vi "macro_Ctrl_LTVUnicycleExecute.vi"() -> ()   [LabVIEW 2019]
uses:
  <vilib>/Rock Robotics/WPI/ThirdParty/JAS_Junk/TrajLib/Trajectory_Library.lvlib
  <vilib>/Rock Robotics/WPI/ThirdParty/JAS_Junk/TrajLib/TypeDef/TRANSLATION2D.ctl
  <vilib>/Rock Robotics/WPI/ThirdParty/JAS_Junk/TrajLib/TypeDef/ROTATION2D.ctl
  <vilib>/Rock Robotics/WPI/ThirdParty/JAS_Junk/TrajLib/TypeDef/POSE2D.ctl
  TypeDef/PathPlannerPathConstraints.ctl
  TypeDef/PathPlannerTrajectoryState.ctl
panel:
  in  "CurrentPose":T1={"TRANSLATION"={"X"=0.0, "Y"=0.0}, "ROTATION"={"VALUE"=0.0, "COS"=1.0, "SIN"=0.0}} {"ROTATION"."SIN" format="%13.4f"; "ROTATION"."COS" format="%13.4f"; "ROTATION"."VALUE" format="%13.4f"; "TRANSLATION"."Y" format="%14.3f"; "TRANSLATION"."X" format="%14.3f"}
  out "Right Speed Dmd M/S":dbl
  out "Left Speed Dmd M/S":dbl
  in  "PathPlannerState":T4={"TimeSeconds"=0.0, "VelocityMPS"=0.0, "AccerationMpsSq"=0.0, "HeadingAngularVelRadPerSec"=0.0, "PositionMeters"={"X"=0.0, "Y"=0.0}, "Heading"={"VALUE"=0.0, "COS"=1.0, "SIN"=0.0}, "TargetHolonomicRotation"={"VALUE"=0.0, "COS"=1.0, "SIN"=0.0}, "CurvatureRadPerMeter"=0.0, "PathPlannerConstraints"={"MaxVelocityMps;"=0.0, "MaxAccelerationMpsSq;"=0.0, "MaxAngularVelRadPsEc;"=0.0, "MaxAngularAccRadPSecSq"=0.0, "Exists"=FALSE}, "DeltaPos"=0.0} {"TargetHolonomicRotation"."SIN" format="%13.4f"; "TargetHolonomicRotation"."COS" format="%13.4f"; "TargetHolonomicRotation"."VALUE" format="%13.4f"; "Heading"."SIN" format="%13.4f"; "Heading"."COS" format="%13.4f"; "Heading"."VALUE" format="%13.4f"; "PositionMeters"."Y" format="%14.3f"; "PositionMeters"."X" format="%14.3f"}
  out "Position Error M":dbl
  out "At Reference":bool
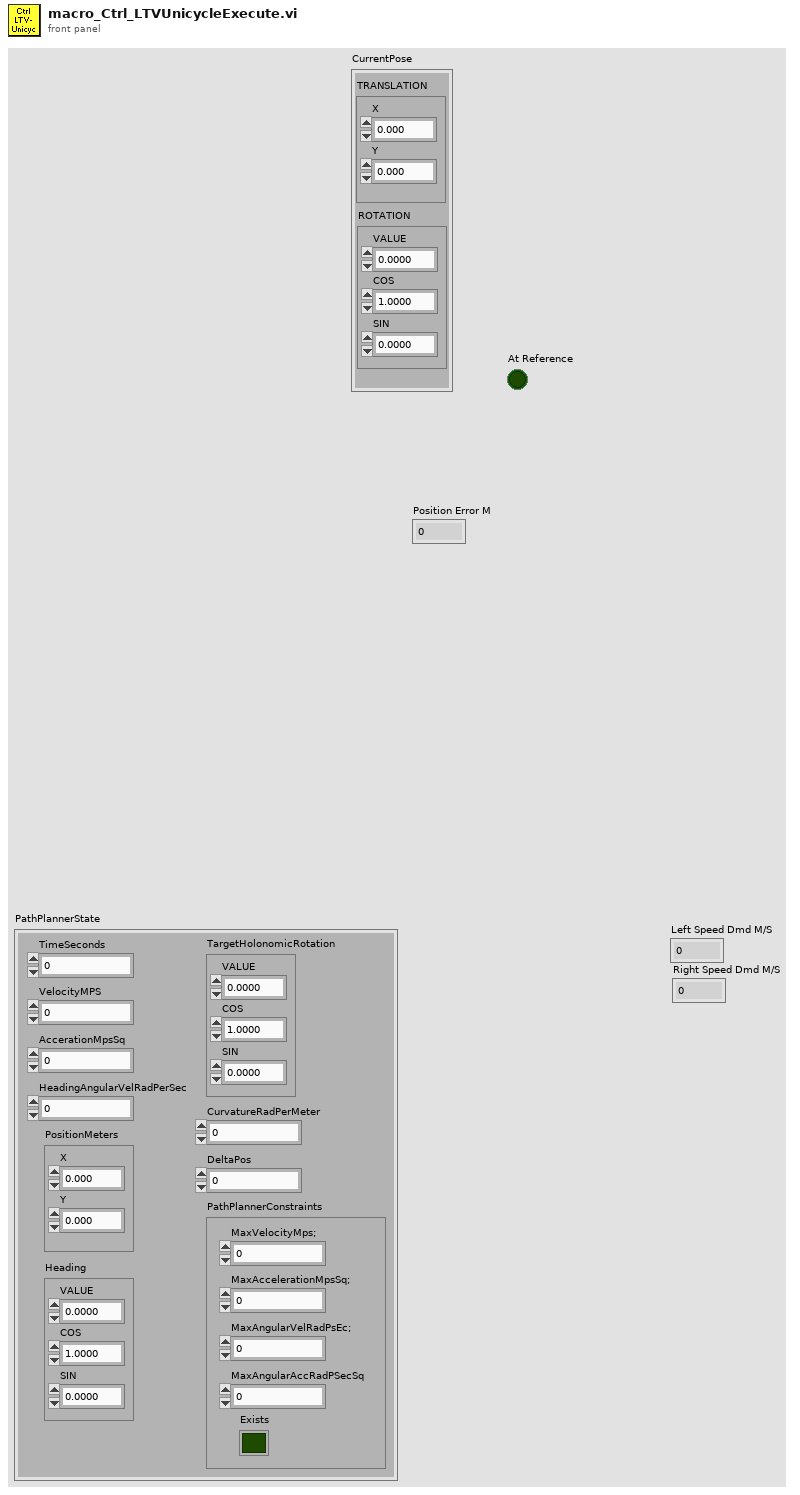
[diagram p1: front panel]
types:
  T1 = typedef "Trajectory_Library.lvlib/POSE2D.ctl" = cluster{"TRANSLATION":T2, "ROTATION":T3}
  T2 = typedef "Trajectory_Library.lvlib/TRANSLATION2D.ctl" = cluster{"X":dbl, "Y":dbl}
  T3 = typedef "Trajectory_Library.lvlib/ROTATION2D.ctl" = cluster{"VALUE":dbl, "COS":dbl, "SIN":dbl}
  T4 = typedef "PathPlannerTrajectoryState.ctl" = cluster{"TimeSeconds":dbl, "VelocityMPS":dbl, "AccerationMpsSq":dbl, "HeadingAngularVelRadPerSec":dbl, "PositionMeters":T2, "Heading":T3, "TargetHolonomicRotation":T3, "CurvatureRadPerMeter":dbl, "PathPlannerConstraints":T5, "DeltaPos":dbl}
  T5 = typedef "PathPlannerPathConstraints.ctl" = cluster{"MaxVelocityMps;":dbl, "MaxAccelerationMpsSq;":dbl, "MaxAngularVelRadPsEc;":dbl, "MaxAngularAccRadPSecSq":dbl, "Exists":bool}
  T6 = typedef "Trajectory_Library.lvlib/LTV_UNICYCLE_CONTROLLER_MODEL_PARAMS.CTL" = cluster{"Max linear ctrl effort M/S":dbl, "Max angular ctrl effort Rad/S":dbl, "Max Heading Meas Tol Rad":dbl, "Max X Pos Meas Tol M":dbl, "Max Y Pos Meas Tol M":dbl, "Max Linear Vel M/S":dbl}
  T7 = typedef "PathPlannerCtrlLTVUnicycleConfig.ctl" = cluster{"Max Wheel Speed M/S":dbl, "Track Width M":dbl, "LTV_Unicycle_Ctrl_Model":T6, "LTV_Unicycle_Ctrl_Tolerance":T8}
  T8 = typedef "Trajectory_Library.lvlib/LTV_UNICYCLE_CONTROLLER_TOLERANCE.CTL" = cluster{"Max Heading Tolerance Rad":dbl, "Max X Tolerance M":dbl, "Max Y Tolerance M":dbl}
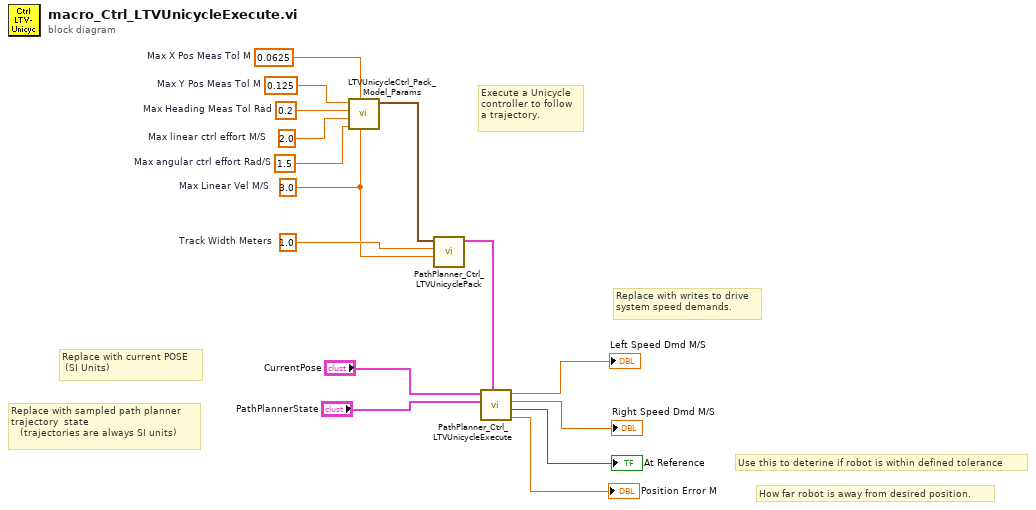
[diagram p0: block diagram]
diagram:
  w2 = 1.0  # Track Width Meters
  w11 = 0.125  # Max Y Pos Meas Tol M
  w12 = 0.2  # Max Heading Meas Tol Rad
  w13 = 2.0  # Max linear ctrl effort M/S
  w14 = 1.5  # Max angular ctrl effort Rad/S
  w15 = 0.0625  # Max X Pos Meas Tol M
  w1 = 3.0  # Max Linear Vel M/S
  # "Execute a Unicycle\ncontroller to follow\na trajectory."
  # "Replace with writes to drive\nsystem speed demands."
  # "Replace with current POSE\n (SI Units)"
  # "Replace with sampled path planner \ntrajectory  state \n   (trajectories are always SI units)"
  # "How far robot is away from desired position."
  # "Use this to deterine if robot is within defined tolerance"
  n1 = call <vilib>:"LTVUnicycleCtrl_Pack_Model_Params.vi"("Max Linear Vel M/S"=w1, "Max X Pos Meas Tol M"=w15, "Max angular ctrl effort Rad/S"=w14, "Max linear ctrl effort M/S"=w13, "Max Heading Meas Tol Rad"=w12, "Max Y Pos Meas Tol M"=w11) -> ("LTV_Unicycle_Ctrl_Model _Params"=w3:T6)  [unwired: 5 in]
  n2 = call "PathPlanner_Ctrl_LTVUnicyclePack.vi"("Max Speed M/S"=w1, "Track Width Meters"=w2, "LTV_Unicycle_Ctrl_Model"=w3) -> ("PathPlanner_Ctrl_LTVUnicycleConfig"=w4:T7)  [unwired: 8 in]
  n3 = call "PathPlanner_Ctrl_LTVUnicycleExecute.vi"("PathPlanner_Ctrl_LTVUnicycle_Config"=w4, "PathPlannerState"="PathPlannerState", "Current Pose SI"="CurrentPose") -> ("Position Error M"=→"Position Error M":dbl, "At Reference"=→"At Reference":bool, "Normalized Right Wheel Dmd M/S"=→"Right Speed Dmd M/S":dbl, "Normalized Left Wheel Dmd M/S"=→"Left Speed Dmd M/S":dbl)  [unwired: 4 in, 1 out]
